vi "TestMain.vi"   [LabVIEW 2020]
uses:
  <vilib>/Neosoft Technologies Inc/Improved Error Dialog/Error Dialog w Copy to Clipboard.lvlib
types:
  T1 = typedef "User-Info.ctl" = cluster{"UserName":string, "Password":string, "Role":T2}
  T2 = typedef "User-Role.ctl" = enum16{"Admin", "Engineer", "Operator"}
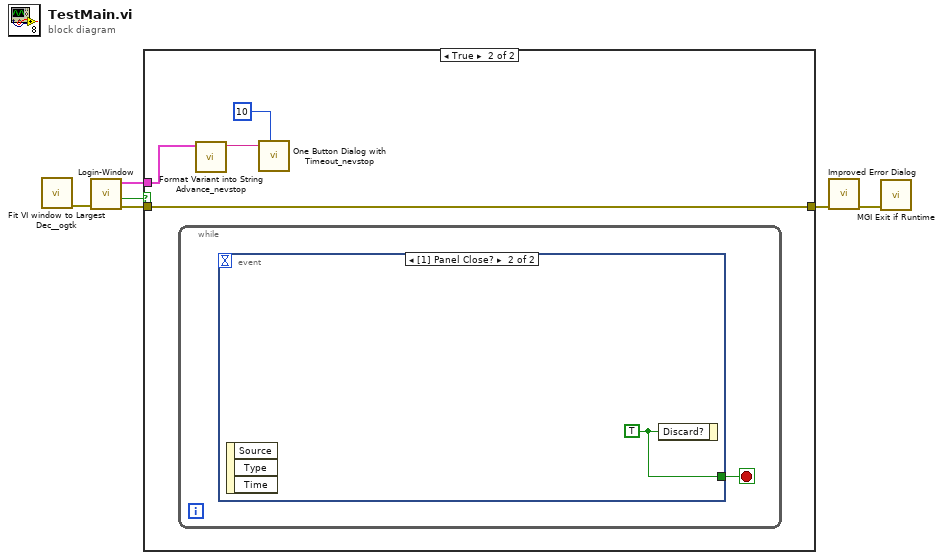
[diagram p0: block diagram]
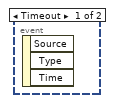
[diagram p3: hidden frame]
diagram:
  n1 = call <userlib>:"Fit VI window to Largest Dec__ogtk.vi"() -> ("error out"=w1:errorcluster)  [unwired: 6 in, 1 out]
  n2 = call "Login-Window.vi"("Error in"=w1) -> ("Error out"=w3:errorcluster, "Valid User"=w5:bool, "User Info"=w4:T1)  [unwired: 8 in]
  n3 = case shown="True" w5 {
    tunnel: w4 -> [_ w11]
    tunnel: w3 -> [w7 w8]
    tunnel: [w7 w8] -> w2
    frame False {
    }
    frame True {
      n4 = while {
        stop <- w12 stop-if-true
        n5 = event shown="[1] Panel Close?" {
          selector: _ -> [_ _]
          dyn-events: _ -> [_ _]
          timeout: _ -> [_ _]
          tunnel: [_ w13] -> w12
          event Timeout {
            n6 = event-data() -> ()  [unwired: 1 in, 3 out]
          }
          event Panel Close? {
            w13 = TRUE ("Discard?")
            n7 = event-data() -> ()  [unwired: 1 in, 3 out]
            n8 = event-data("Discard?"=w13) -> ()  [unwired: 1 in, 1 out]
          }
        }
      }
      n9 = call <userlib>:"Format Variant into String Advance_nevstop.vi"("Variant"=w11) -> ("Data"=w10:string)  [unwired: 8 in, 2 out]
      n10 = call <userlib>:"One Button Dialog with Timeout_nevstop.vi"("message"=w10, "Btn Timeout(-1 s)"=10) -> ()  [unwired: 7 in, 1 out]
    }
  }
  n11 = call <vilib>:"Improved Error Dialog.vi"("error in (no error)"=w2) -> ("error out"=w6:errorcluster)  [unwired: 10 in]
  n12 = call <userlib>:"MGI Exit if Runtime.vi"("Error In (Dependency Only)"=w6) -> ()  [unwired: 11 in]
